vi "Query Zoom Window Time Scale.vi"(8 "error in (no error)":errorcluster, 11 "VISA resource name":refnum<visa-resource-name>) -> (0 "error out":errorcluster, 2 "Current Time Scale":dbl, 3 "VISA resource name out":refnum<visa-resource-name>)   [LabVIEW 2017, in "Tektronix TDS 200 1000 2000 Series.lvlib"]
doc: "Queries the zoom window current time scale.\n\n<B>Note(s):</b>\nAvailable on TBS1000B-EDU and TBS1000B series only."
uses:
  Tektronix TDS 200 1000 2000 Series.lvlib
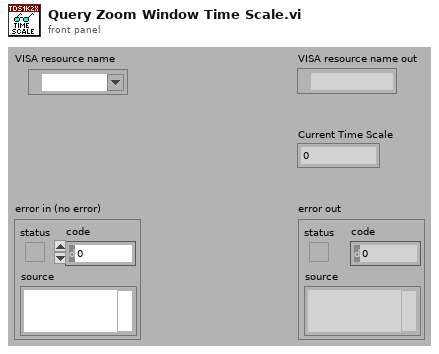
[diagram p1: front panel]
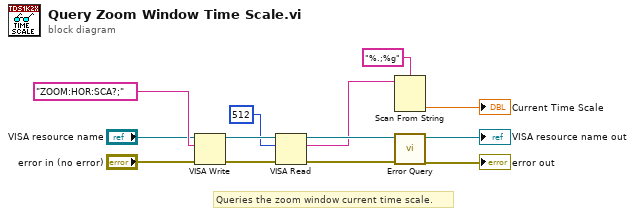
[diagram p0: block diagram]
diagram:
  # "Queries the zoom window current time scale."
  n1 = VISA Write(VISA resource name="VISA resource name", write buffer="ZOOM:HOR:SCA?;", error in (no error)="error in (no error)") -> (VISA resource name out=w8:refnum<visa-resource-name>, error out=w7:errorcluster)  [unwired: 1 out]
  n2 = VISA Read(VISA resource name=w8, byte count=u32 512, error in (no error)=w7) -> (VISA resource name out=w6:refnum<visa-resource-name>, read buffer=w2:string, error out=w5:errorcluster)  [unwired: 1 out]
  n3 = Scan From String(format string="%.;%g", input string=w2) -> (output 1=→"Current Time Scale":dbl)  [unwired: 2 in, 4 out]
  n4 = call "Error Query.vi"("error in (no error)"=w5, "VISA resource name"=w6) -> ("error out"=→"error out":errorcluster, "VISA resource name out"=→"VISA resource name out":refnum<visa-resource-name>)  [unwired: 8 out]
